vi "RD_MatchScore.vi"(10 "name":string="LogMatchScore.txt", 11 "base path":path=path "C:/Users/user/Desktop/SICK-Ranger3/screwDetection/LT") -> (2 "R_Match_Score":dbl, 3 "L_Match_Score":dbl)   [LabVIEW 2019]
uses:
  <vilib>/regexp/Match Regular Expression.xnode
panel:
  out "RawData":string[](array[string])
  out "appended path":path
  out "text":string
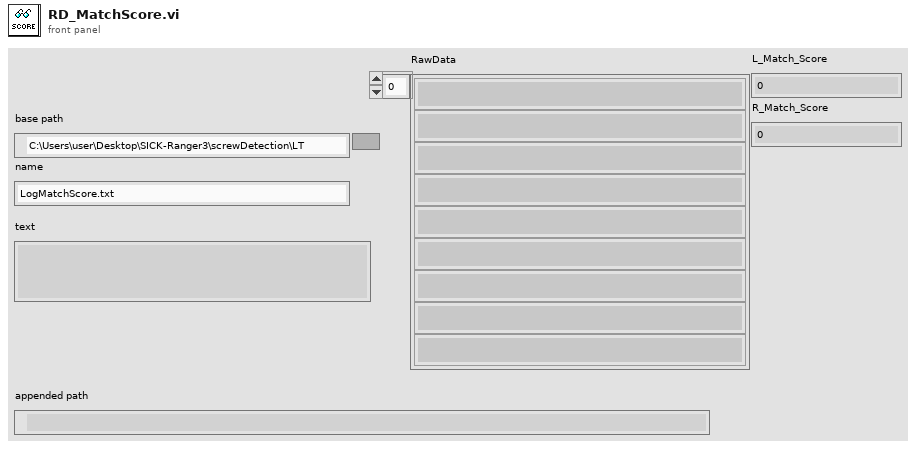
[diagram p1: front panel]
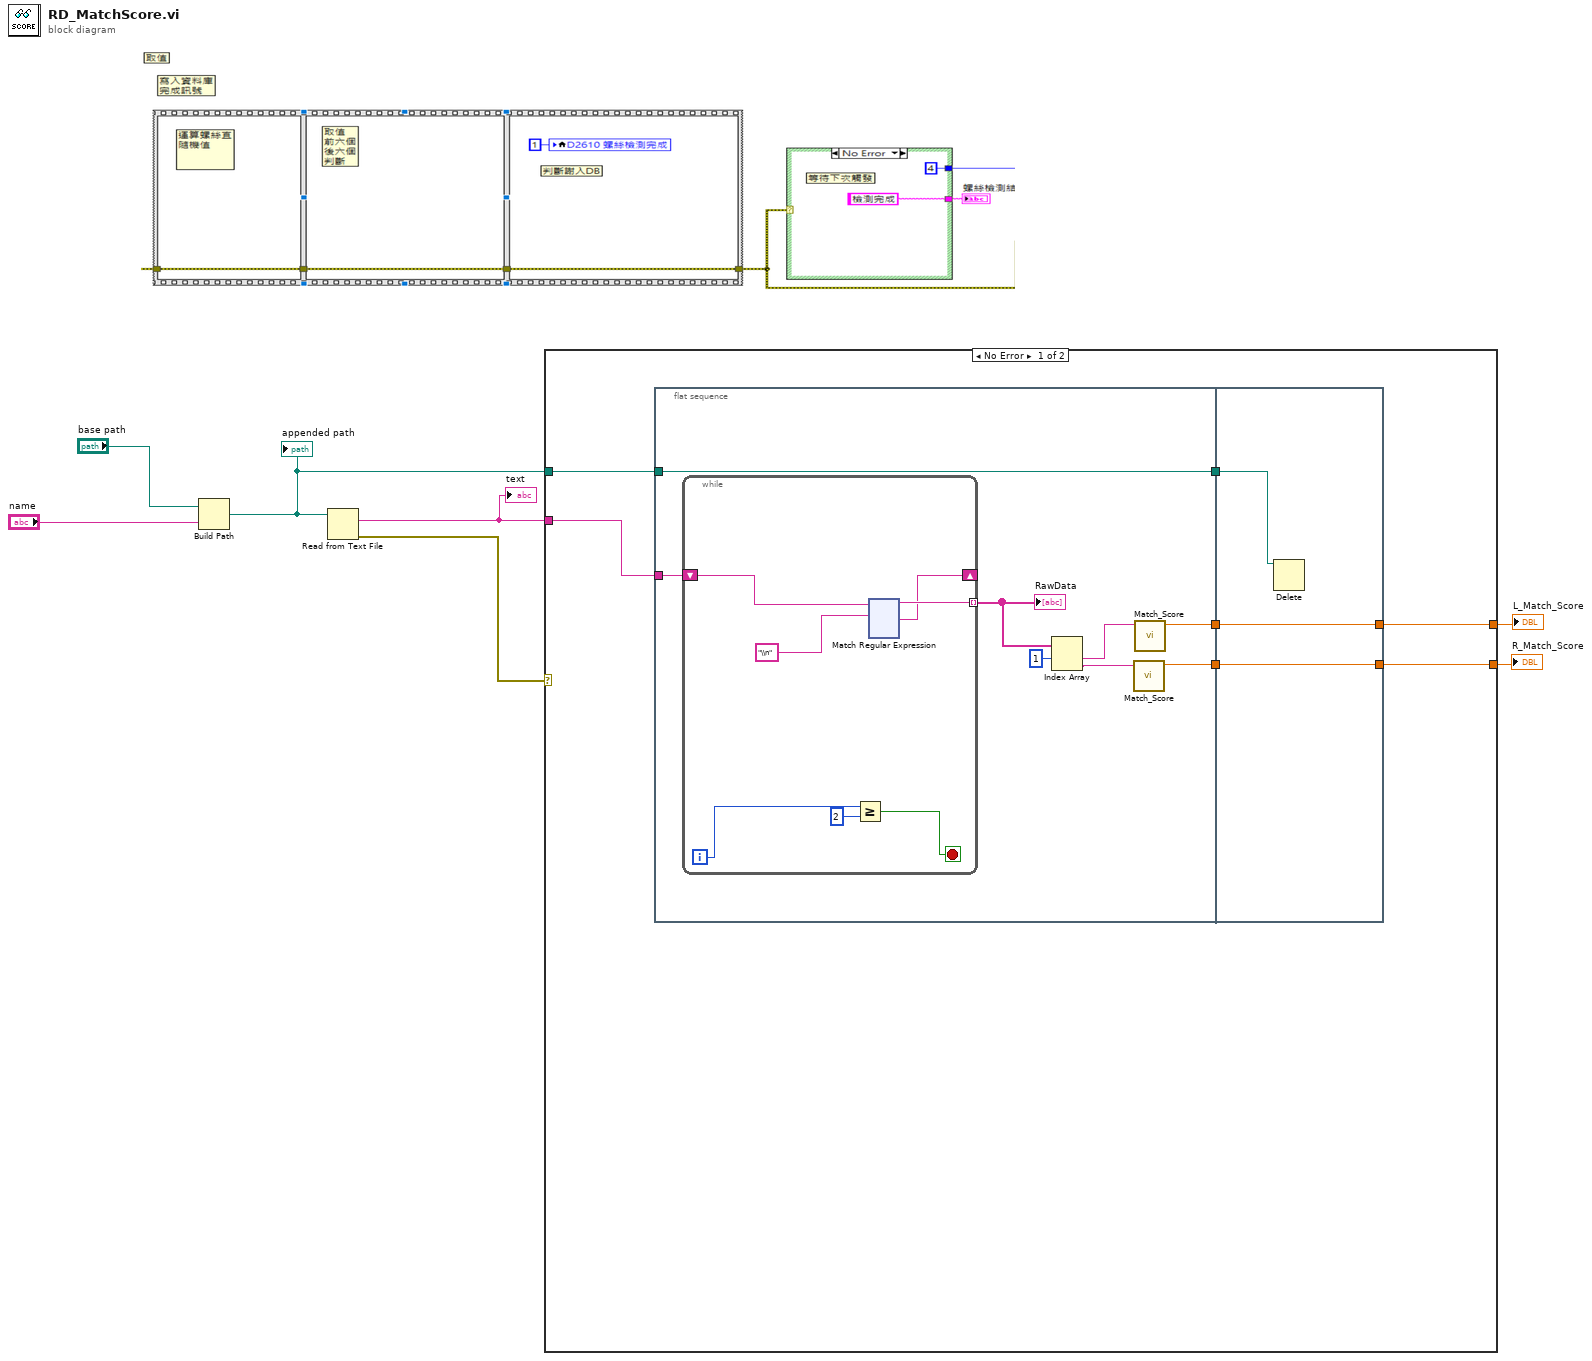
[diagram p0: block diagram]
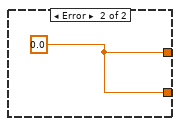
[diagram p2: hidden frame]
diagram:
  n1 = Build Path(base path="base path", name or relative path="name") -> (appended path=w1:path)
  "appended path" <- w1
  n2 = Read from Text File(file (use dialog)=w1) -> (text=w6:string, error out=w7:errorcluster)  [unwired: 3 in, 2 out]
  "text" <- w6
  n3 = case shown="No Error" w7 {
    tunnel: w6 -> [w14 _]
    tunnel: [w13 w147] -> w3
    tunnel: [w12 w147] -> w2
    tunnel: w1 -> [w8 _]
    frame No Error {
      n4 = flat-sequence {
        tunnel: w14 -> [w22]
        tunnel: [w17] -> w11
        tunnel: [w16] -> w10
        tunnel: [w15] -> w9
        tunnel: w8 -> [w15]
        tunnel: [w145] -> w12
        tunnel: [w146] -> w13
        tunnel: w11 -> [w146]
        tunnel: w10 -> [w145]
        tunnel: w9 -> [w144]
        frame #0 {
          n5 = while {
            shift-right: [w26] -> _
            shift-left: w22 -> [w29]
            tunnel: [w27] -> w21 mode=indexing
            i -> [w25]
            stop <- w23 stop-if-true
            n6 = Greater Or Equal?(x=w25, y=2) -> (x >= y?=w23:bool)
            n7 = xnode "Match Regular Expression"("input string"=w29, "regular expression"="\\n") -> ("before match"=w27:string, "after match"=w26:string)  [unwired: 4 in, 3 out]
          }
          "RawData" <- w21
          n8 = Index Array(array=w21, index #1=1 ("index")) -> (element #1=w19:string, element #2=w18:string)  [unwired: 1 in]
          n9 = call "Match_Score.vi"("before match in"=w18) -> ("number"=w16:dbl)  [unwired: 10 in]
          n10 = call "Match_Score.vi"("before match in"=w19) -> ("number"=w17:dbl)  [unwired: 10 in]
        }
        frame #1 {
          n11 = Delete(path (use dialog)=w144) -> ()  [unwired: 4 in, 3 out]
        }
      }
    }
    frame Error {
      w147 = 0.0 ("number")
    }
  }
  "R_Match_Score" <- w2
  "L_Match_Score" <- w3
